vi "Test Set Range on Control.vi"() -> ()   [LabVIEW 2012]
uses:
  Reusable/General/Atmospheric/Atmospheric Library.lvlib
  Reusable/General/Temperature/Temperature.lvlib
panel:
  out "T out":dbl
  out "Vout":sgl
  in  "T":dbl
  out "x/y":dbl
  out "es":dbl
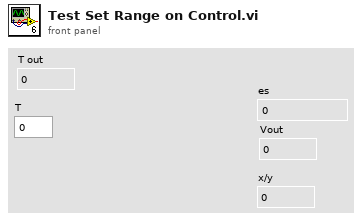
[diagram p1: front panel]
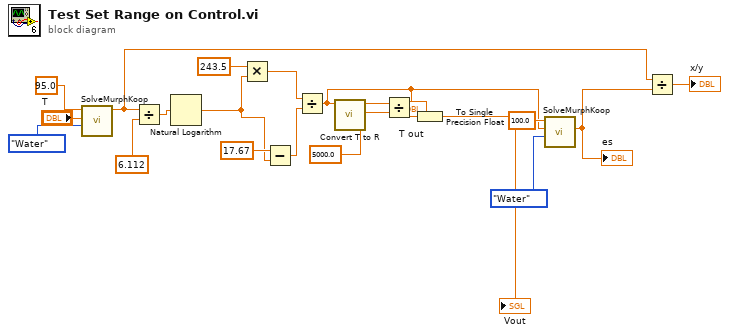
[diagram p0: block diagram]
diagram:
  n1 = call "SolveMurphKoop.vi"("Type"=enum16{"Ice", "Water"}."Water", "T"="T", "RH"=95.0) -> ("e"=w6:dbl)  [unwired: 5 in, 3 out]
  n2 = Divide(x=w6, y=6.112) -> (x/y=w15:dbl)
  n3 = Natural Logarithm(1:w15) -> (0:w14:dbl)
  n4 = Multiply(x=243.5, y=w14) -> (x*y=w13:dbl)
  n5 = Subtract(x=17.67, y=w14) -> (x-y=w12:dbl)
  n6 = Divide(x=w13, y=w12) -> (x/y=w1:dbl)
  "T out" <- w1
  n7 = call "Convert T to R.vi"("T"=w1) -> ("R"=w11:dbl)  [unwired: 10 in]
  n8 = Divide(x=w11, y=5000.0) -> (x/y=w9:dbl)
  n9 = To Single Precision Float(number=w9) -> (single precision float=→"Vout":sgl)
  n10 = call "SolveMurphKoop.vi"("Type"=enum16{"Ice", "Water"}."Water", "T"=w1, "RH"=100.0) -> ("es"=w7:dbl)  [unwired: 5 in, 3 out]
  "es" <- w7
  n11 = Divide(x=w6, y=w7) -> (x/y=→"x/y":dbl)
